vi "Actor Core.vi"(8 "error in":errorcluster, 11 "Acquisition UI in":refnum<class "Acquisition UI.lvclass">) -> (0 "error out":errorcluster, 3 "Actor out":refnum<class "Actor.lvclass">)   [LabVIEW 2018, in "Acquisition UI.lvlib" / "Acquisition UI.lvclass"]
doc: "(<B>Filename</B>: Actor Framework.lvlib:Actor.lvclass:Actor Core.vi)\n\nReceives messages to the actor, reacts to them, and initiates any error handling that may shut the actor down.\n\nDescendant classes may override this VI to append parallel tasks for the actor to complete while it handles messages. Overrides use the Call Parent Method node."
uses:
  Acquisition UI.lvclass
  C:/Program Files (x86)/National Instruments/LabVIEW 2018/vi.lib/ActorFramework/Actor/Actor.lvclass
  <vilib>/ActorFramework/Actor/Actor.lvclass
  Acquisition/Acquisition/Acquisition.lvclass
  <vilib>/ActorFramework/Actor/Actor.lvclass/Actor.ctl
  <vilib>/ActorFramework/Message Enqueuer/Message Enqueuer.lvclass/Message Enqueuer.ctl
  Acquisition UI.lvclass/Acquisition UI.ctl
  <vilib>/ActorFramework/Message Enqueuer/Init from Existing Queue.vi
  <vilib>/ActorFramework/Message Enqueuer/Enqueue.vi
  Acquisition/Acquisition Messages/Start Acquisition Msg/Start Acquisition Msg.lvclass
  C:/Program Files (x86)/National Instruments/LabVIEW 2018/vi.lib/ActorFramework/Message/Message.lvclass
  Acquisition/Acquisition Messages/Stop Acquisition Msg/Stop Acquisition Msg.lvclass
  <vilib>/ActorFramework/Stop Msg/Stop Msg.lvclass
  <vilib>/ActorFramework/Message Priority Queue/Priority Enqueue.vi
  <vilib>/ActorFramework/Message Enqueuer/Message Enqueuer.lvclass
panel:
  out "Data":waveform(dbl)[](graph)
  in  "Stop Acquistion":bool
  in  "Start Acquisition":bool
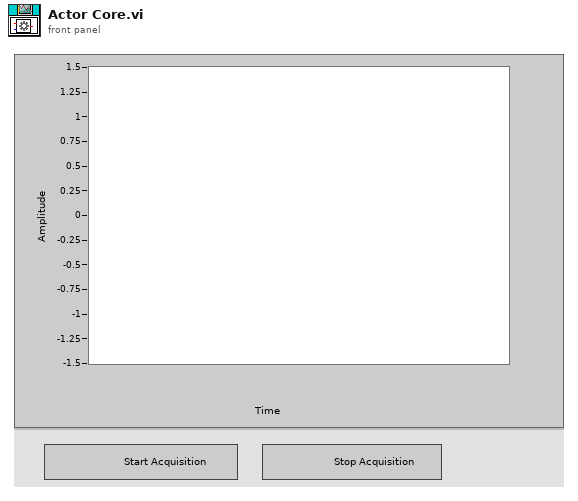
[diagram p1: front panel]
types:
  T1 = typedef "Acquisition UI.lvlib/Acquisition UI.lvclass/Helper Loop Events--cluster.ctl" = cluster{"Display Graph Data":refnum<user-event>, "Stop Helper Loop":refnum<user-event>}
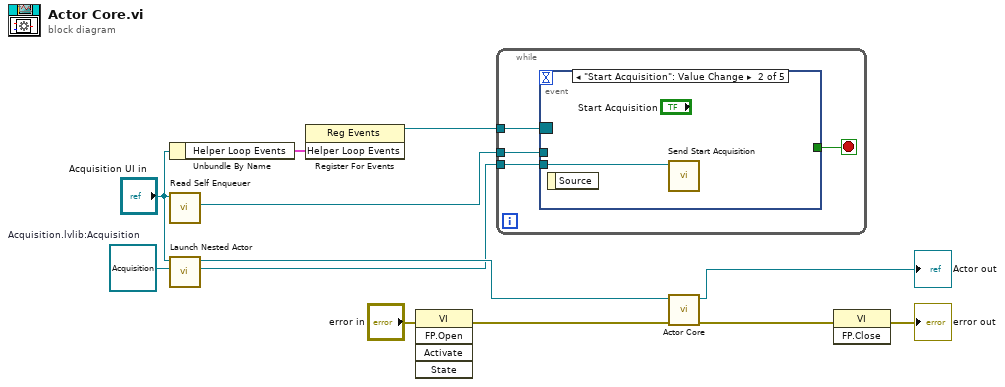
[diagram p0: block diagram]
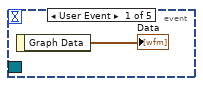
[diagram p2: hidden frame]
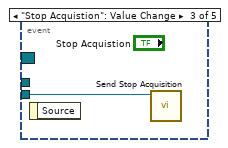
[diagram p3: hidden frame]
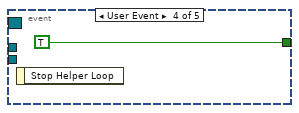
[diagram p4: hidden frame]
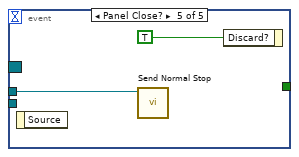
[diagram p5: hidden frame]
diagram:
  w3 = refnum<class "Acquisition.lvclass"> refnum  # Acquisition.lvlib:Acquisition
  n1 = Unbundle By Name("Acquisition UI in") -> ("Helper Loop Events"=w10:T1)
  n2 = call <vilib>:"Read Self Enqueuer.vi"("Actor"="Acquisition UI in") -> ("Self Enqueuer"=w5:refnum<class "Message Enqueuer.lvclass">)  [unwired: 10 in]
  n3 = call <vilib>:"Launch Nested Actor.vi"("Nested Actor"=w3, "Caller Actor in"="Acquisition UI in") -> ("Nested Actor's Enqueuer"=w1:refnum<class "Message Enqueuer.lvclass">, "Caller Actor out"=w2:refnum<class "Acquisition UI.lvclass">)  [unwired: 7 in, 1 out]
  n4 = register-events(w10) -> (reference out=w11:refnum<event-registration>)  [unwired: 2 in, 1 out]
  n5 = invoke class="VI" method="FP.Open"(error in="error in") -> (error out=w8:errorcluster)  [unwired: 4 in, 4 out]
  n6 = while {
    tunnel: w11 -> [w16]
    tunnel: w5 -> [w14]
    tunnel: w1 -> [w13]
    stop <- w15 stop-if-true
    n7 = event shown="[1] \"Start Acquisition\": Value Change" {
      selector: w16 -> [_ _ _ _ _]
      dyn-events: _ -> [_ _ _ _ _]
      timeout: _ -> [_ _ _ _ _]
      tunnel: [_ _ _ TRUE _] -> w15
      tunnel: w14 -> [_ _ _ _ w21]
      tunnel: w13 -> [_ w18 w19 _ _]
      event User Event {
        n8 = event-data() -> ("Graph Data"=→"Data":waveform(dbl)[])  [unwired: 1 in]
      }
      event "Start Acquisition": Value Change {
        n9 = event-data() -> ()  [unwired: 1 in, 1 out]
        n10 = call "Send Start Acquisition.vi"("Message Enqueuer"=w18) -> ()  [unwired: 9 in, 2 out]
      }
      event "Stop Acquistion": Value Change {
        n11 = event-data() -> ()  [unwired: 1 in, 1 out]
        n12 = call "Send Stop Acquisition.vi"("Message Enqueuer"=w19) -> ()  [unwired: 9 in, 2 out]
      }
      event User Event {
        n13 = event-data() -> ()  [unwired: 1 in, 1 out]
      }
      event Panel Close? {
        n14 = event-data() -> ()  [unwired: 1 in, 1 out]
        n15 = call <vilib>:"Send Normal Stop.vi"("Message Enqueuer"=w21) -> ()  [unwired: 10 in, 1 out]
        n16 = event-data("Discard?"=TRUE) -> ()  [unwired: 1 in, 1 out]
      }
    }
  }
  n17 = call-parent "Actor Core.vi"("error in"=w8, "Actor in"=w2) -> ("error out"=w7:errorcluster, "Actor out"=→"Actor out":refnum<class "Actor.lvclass">)  [unwired: 8 in]
  n18 = invoke class="VI" method="FP.Close"(error in=w7) -> (error out=→"error out":errorcluster)  [unwired: 2 in, 2 out]
